vi "NI VeriStand - Get Loop Flags.vi"(8 "error in (no error)":errorcluster, 11 "Item Ref in":T2 format="%.0x") -> (0 "error out":errorcluster, 2 "Loop Flags":T1, 3 "Item Ref out":T2 format="%.0x")   [LabVIEW 2020, in "Custom Device API.lvlib"]
doc: "Returns the flags that determine what steps the custom device skips."
uses:
  <vilib>/NI VeriStand/Custom Device API/Custom Device API.lvlib
  <vilib>/NI VeriStand/Custom Device API/Custom Device Item Ref.ctl
  <vilib>/NI VeriStand/Custom Device API/Custom Device Loop Flags.ctl
  df5b1ffc-b8f5-47c1-b762-da9e36ced45e.vi
  <vilib>/NI VeriStand/Custom Device API/Custom Device Offline Path.vi
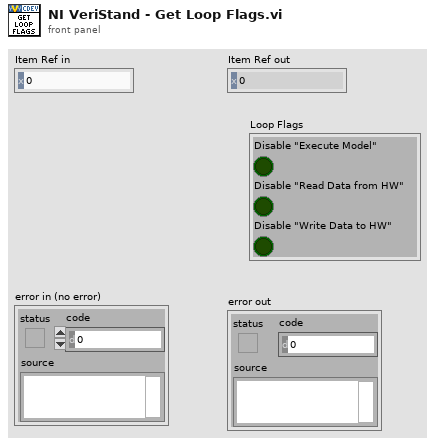
[diagram p1: front panel]
types:
  T1 = typedef "Custom Device API.lvlib/Custom Device Loop Flags.ctl" = cluster{"Disable \"Execute Model\"":bool, "Disable \"Read Data from HW\"":bool, "Disable \"Write Data to HW\"":bool}
  T2 = typedef "Custom Device API.lvlib/Custom Device Item Ref.ctl" = u64
  T3 = typedef "Custom Devices Storage.lvlib/Loop Flags.ctl" = cluster{"Disable \"Execute Model\"":bool, "Disable \"Read Data from HW\"":bool, "Disable \"Write Data to HW\"":bool}
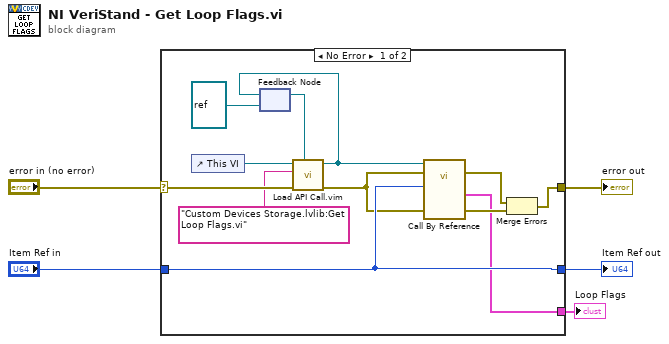
[diagram p0: block diagram]
diagram:
  n1 = case shown="No Error" "error in (no error)" {
    selector: "error in (no error)" -> [w11 w19]
    tunnel: [w17 w19] -> w5
    tunnel: "Item Ref in" -> [w15 w18]
    tunnel: [w15 w18] -> w2
    tunnel: [w14 _] -> w1
    frame No Error {
      n2 = control-ref of="This VI"() -> (w12:refnum<vi>)
      n3 = feedback #1(refnum<vi> refnum ("type specifier VI Refnum (for type only)")) -> (w13:refnum<vi>)
      n4 = call "Load API Call.vim"("VI reference in"=w13, "error in (no error)"=w11, "VI qualified name"="Custom Devices Storage.lvlib:Get Loop Flags.vi", "Caller VI ref"=w12) -> ("error out"=w10:errorcluster, "VI reference"=w9:refnum<vi>)  [unwired: 6 in]
      n5 = feedback-in #1(w9) -> ()
      n6 = call-by-ref "?"(reference=w9, error in=w10, 8:"error in (no error)"=w10, "Item Ref in"=w15) -> (error out=w6:errorcluster, 0:"error out"=w16:errorcluster, "Loop Flags"=w14:T3)  [unwired: 7 in, 2 out]
      n7 = Merge Errors(w6, w16) -> (w17:errorcluster)
    }
    frame Error {
    }
  }
  "Item Ref out" <- w2
  "error out" <- w5
  "Loop Flags" <- w1
